vi "Configure Mediator.vi"(9 "Framework Instance Alias":string, 10 "Event Log Instance":refnum<class "LoggerReference.lvclass">, 11 "Mediator in":refnum<class "IMediator.lvclass">) -> (3 "Mediator out":refnum<class "IMediator.lvclass">)   [LabVIEW 2017, in "IMediator.lvlib" / "IMediator.lvclass"]
uses:
  <vilib>/gpm_packages/@cs/mva-core/Source/IMediator/IMediator/IMediator.lvclass
  <vilib>/gpm_packages/@cs/event-logger/Source/Composed Log/LoggerReference/LoggerReference.lvclass
  <vilib>/gpm_packages/@cs/mva-core/Source/IMediator/IMediator/IMediator.lvclass/IMediator.ctl
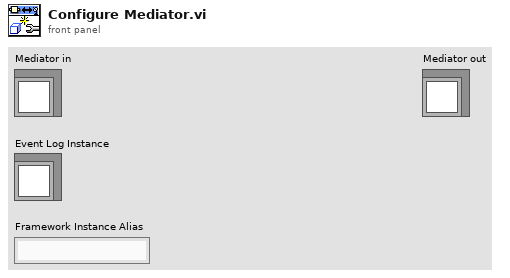
[diagram p1: front panel]
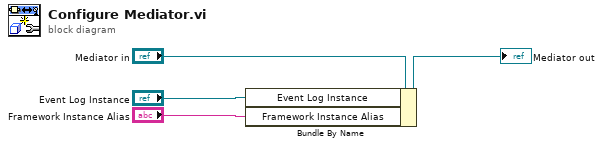
[diagram p0: block diagram]
diagram:
  n1 = Bundle By Name(cluster="Mediator in", "Event Log Instance"="Event Log Instance", "Framework Instance Alias"="Framework Instance Alias") -> (→"Mediator out":refnum<class "IMediator.lvclass">)
